vi "AssertNotRefnum.vi"(7 "Message (\"\")":string, 8 "error in (no error)":errorcluster, 10 "Refnum":variant) -> (0 "error out":errorcluster)   [LabVIEW 2017, in "Assertion.lvlib"]
doc: "Asserts that a variable is not a valid refnum. Does nothing if an error occurred before this node runs. Returns an error if the assertion failed. Optionally adds a message to the error message if the assertion failed."
uses:
  Assertion.lvlib
  Constraint/IsRefnum/IsRefnum.lvclass
  Constraint/UnaryOperator/UnaryOperator.lvclass
  Constraint/LogicalNot/LogicalNot.lvclass
  C:/Users/de200256/Code/neuperger/lvunit/Constraint/Constraint/Constraint.lvclass
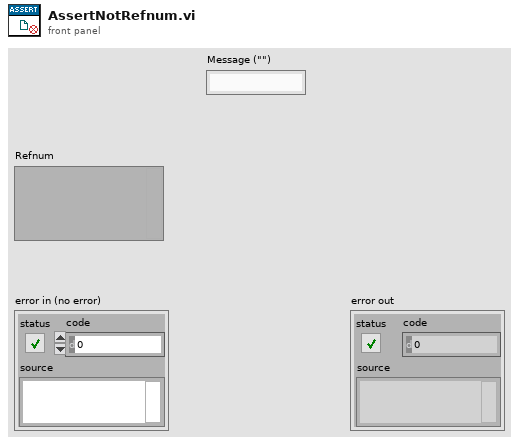
[diagram p1: front panel]
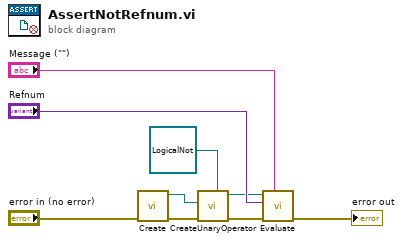
[diagram p0: block diagram]
diagram:
  n1 = call "Create.vi"("error in (no error)"="error in (no error)") -> ("error out"=w8:errorcluster, "IsRefnum"=w4:refnum<class "IsRefnum.lvclass">)  [unwired: 9 in]
  n2 = call-dynamic "CreateUnaryOperator.vi"("UnaryOperator In"=refnum<class "LogicalNot.lvclass"> refnum, "error in (no error)"=w8, "Constraint"=w4) -> ("error out"=w5:errorcluster, "UnaryOperator"=w2:refnum<class "UnaryOperator.lvclass">)  [unwired: 7 in]
  n3 = call-dynamic "Evaluate.vi"("Message (\"\")"="Message (\"\")", "error in (no error)"=w5, "Actual"="Refnum", "Constraint in"=w2) -> ("error out"=→"error out":errorcluster)  [unwired: 6 in, 1 out]
